vi "test Value to String to Value (Boolean).vi"(8 "error in":errorcluster, 11 "TestCase in":refnum<class "SharedUtilities.lvclass">) -> (0 "error out":errorcluster, 3 "TestCase out":refnum<class "SharedUtilities.lvclass">)   [LabVIEW 2020, in "SharedUtilities.lvclass"]
uses:
  SharedUtilities.lvclass
  a53efd5e-1b89-4488-9cb0-ebdcaa892606.vi
  e7dd0ea7-1b51-4b32-9c58-6851ae4c1315.vi
  0f61251e-6bce-40bc-9127-ed727464e5d8.vi
  4657b86e-0f3a-47b0-a768-c094f0f21e47.vi
  <vilib>/addons/_JKI Toolkits/VI Tester/TestCase.llb/TestCase.lvclass
  C:/Program Files (x86)/National Instruments/LabVIEW 2020/vi.lib/addons/_JKI Toolkits/VI Tester/TestCase.llb/TestCase.lvclass
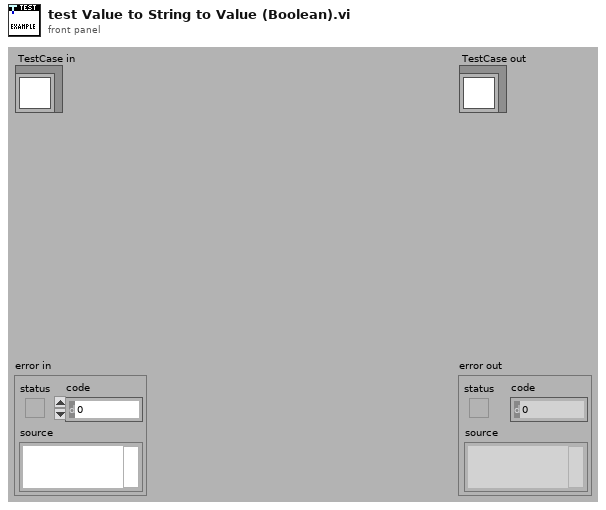
[diagram p1: front panel]
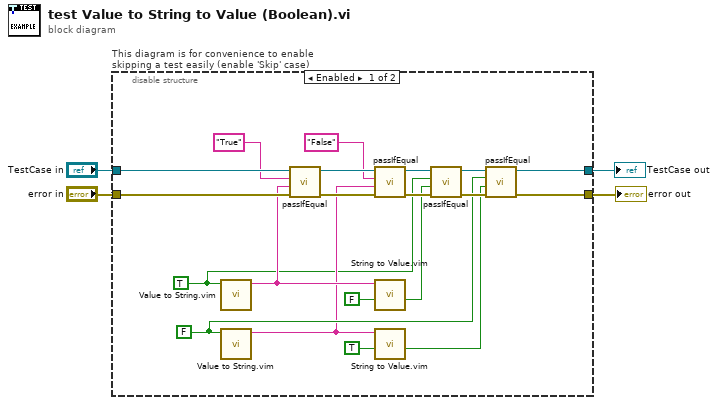
[diagram p0: block diagram]
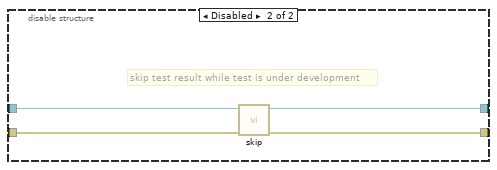
[diagram p2: hidden frame]
diagram:
  n1 = disable-structure "This diagram is for convenience to enable skipping a test easily (enable 'Skip' case)" shown="Enabled" {
    disable-tunnel: "TestCase in" -> [w14 w28]
    disable-tunnel: [w18 w26] -> w1
    disable-tunnel: [w17 w27] -> w3
    disable-tunnel: "error in" -> [w13 w25]
    frame Enabled {
      w12 = FALSE
      w5 = TRUE
      n2 = call "Value to String.vim"("value"=w5) -> ("string"=w9:string)  [unwired: 10 in]
      n3 = call "Value to String.vim"("value"=w12) -> ("string"=w6:string)  [unwired: 10 in]
      n4 = call-dynamic "passIfEqual.vi"("error in (no error)"=w13, "y"=w9, "x"="True" ("string"), "TestCase in"=w14) -> ("error out"=w16:errorcluster, "TestCase out"=w15:refnum<class "SharedUtilities.lvclass">)  [unwired: 6 in]
      n5 = call-dynamic "passIfEqual.vi"("error in (no error)"=w16, "y"=w6, "x"="False" ("string"), "TestCase in"=w15) -> ("error out"=w24:errorcluster, "TestCase out"=w23:refnum<class "SharedUtilities.lvclass">)  [unwired: 6 in]
      n6 = call "String to Value.vim"("default"=FALSE, "string"=w9) -> ("value"=w20:bool)  [unwired: 9 in]
      n7 = call "String to Value.vim"("default"=TRUE, "string"=w6) -> ("value"=w19:bool)  [unwired: 9 in]
      n8 = call-dynamic "passIfEqual.vi"("error in (no error)"=w24, "y"=w20, "x"=w5, "TestCase in"=w23) -> ("error out"=w22:errorcluster, "TestCase out"=w21:refnum<class "SharedUtilities.lvclass">)  [unwired: 6 in]
      n9 = call-dynamic "passIfEqual.vi"("error in (no error)"=w22, "y"=w19, "x"=w12, "TestCase in"=w21) -> ("error out"=w17:errorcluster, "TestCase out"=w18:refnum<class "SharedUtilities.lvclass">)  [unwired: 6 in]
    }
    frame Disabled {
      # "skip test result while test is under development"
      n10 = call <vilib>:"skip.vi"("error in (no error)"=w25, "TestCase in"=w28) -> ("error out"=w27:errorcluster, "TestCase out"=w26:refnum<class "SharedUtilities.lvclass">)  [unwired: 8 in]
    }
  }
  "error out" <- w3
  "TestCase out" <- w1
